vi "runtest format template keys.vi"(0 "Connection Refnum":T11, 1 "POST (empty)":T10, 3 "User Action (Run)":enum16{"Run", "Repeat"}(ring), 5 "Test Sequence ID":string, 9 "Fields / Results":T8, 11 "error in (no error)":errorcluster, 12 "Timer":u32, 13 "User/Station":T1, 14 "Run Permissions":T9) -> (4 "Connection Refnum":T11, 10 "Template Keys":T10, 15 "error out":errorcluster)   [LabVIEW 2011]
uses:
  Addons/internet/utils/keyedarr.llb/Keyed Array.ctl
  SI.LIB/ODBC/SQL Controls/Connection Refnum.ctl
  server/database/Fields/Field Record.ctl
  server/database/Fields/Field DataTypes.ctl
  server/database/Fields/Field NextItem.ctl
  tests/Test Output.ctl
  runtest User - Station.ctl
  server/database/Stations/Instruments/Instrument Record.ctl
  server/database/Stations/Step Associations/Step Association Record.ctl
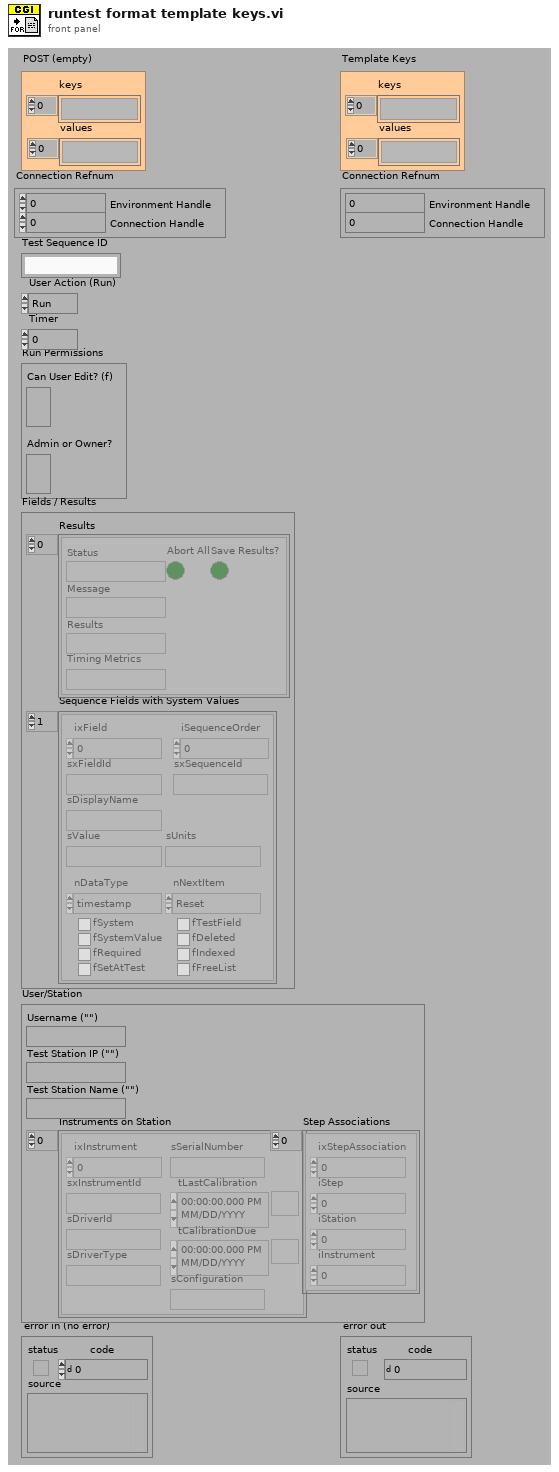
[diagram p1: front panel]
types:
  T1 = typedef "runtest User - Station.ctl" = cluster{"Username (\"\")":string, "Test Station IP (\"\")":string, "Test Station Name (\"\")":string, "Instruments on Station":T2[], "Step Associations":T3[]}
  T2 = typedef "Instrument Record.ctl" = cluster{"ixInstrument":i32, "sxInstrumentId":string, "sDriverId":string, "sDriverType":string, "sSerialNumber":string, "tLastCalibration":timestamp, "tCalibrationDue":timestamp, "sConfiguration":string}
  T3 = typedef "Step Association Record.ctl" = cluster{"ixStepAssociation":i32, "iStep":i32, "iStation":i32, "iInstrument":i32}
  T4 = typedef "Field Record.ctl" = cluster{"ixField":i32, "iSequenceOrder":i32, "sxFieldId":string, "sxSequenceId":string, "sDisplayName":string, "sValue":string, "sUnits":string, "nDataType":T5, "nNextItem":T6, "fSystem":bool, "fSystemValue":bool, "fRequired":bool, "fSetAtTest":bool, "fTestField":bool, "fDeleted":bool, "fIndexed":bool, "fFreeList":bool}
  T5 = typedef "Field DataTypes.ctl" = enum32{"text", "numeric", "list", "timestamp", "boolean"}
  T6 = typedef "Field NextItem.ctl" = enum32{"Reset", "Retain", "Auto-Increment"}
  T7 = typedef "Test Output.ctl" = cluster{"Status":string, "Message":string, "Results":string, "Abort All":bool, "Save Results?":bool, "Timing Metrics":string}
  T8 = cluster{"Sequence Fields with System Values":T4[], "Results":T7[]}
  T9 = cluster{"Can User Edit? (f)":bool, "Admin or Owner?":bool}
  T10 = typedef "Keyed Array.ctl" = cluster{"keys":string[], "values":string[]}
  T11 = typedef "Connection Refnum.ctl" = cluster{"Environment Handle":i32, "Connection Handle":i32}
  T12 = typedef "Sequence Record.ctl" = cluster{"ixSequence":i32, "sxSequenceId":string, "sDescription":string, "sCreator":string, "tCreationDate":timestamp, "sModifier":string, "tModifiedDate":timestamp, "fApproved":bool, "fSpartanSetsSN":bool, "fOverwriteData":bool, "fStopOnFail":bool, "fDisableQuickMode":bool, "fPartialExecution":bool, "fAutoNextItem":bool, "fDoNotPrintOnFail":bool}
  T13 = typedef "Step Record.ctl" = cluster{"ixStep":i32, "sxSequenceId":string, "sxTestId":string, "iIndex":i32, "iRepeat":i32, "iQuickMode":i32, "sTag":string, "sDatasheetsCSV":string, "bConfiguration":string}
  T14 = typedef "Test Record.ctl" = cluster{"ixTest":i32, "sxTestId":string, "sVersion":string, "sDriverTypes":string[], "sDescription":string, "iQuickMode":i32}
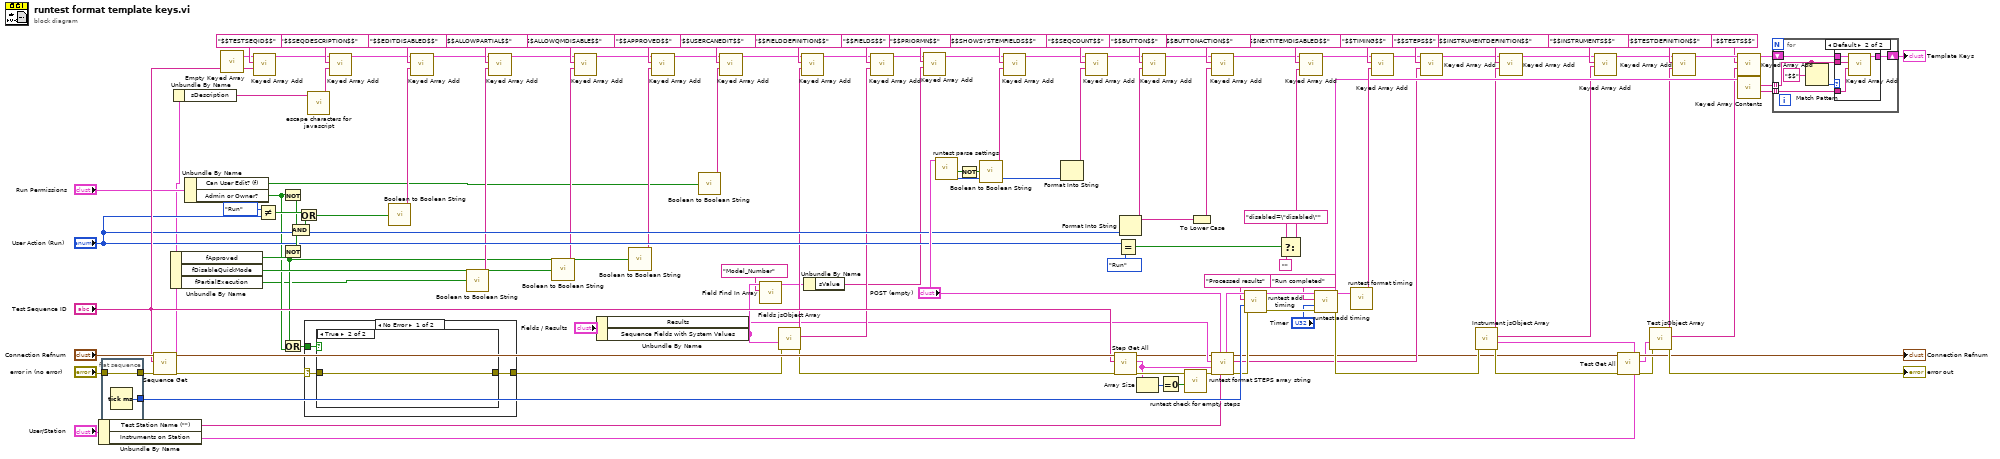
[diagram p0: block diagram]
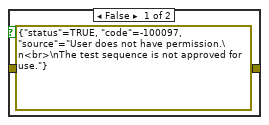
[diagram p2: hidden frame]
diagram:
  n1 = Unbundle By Name("User/Station") -> ("Test Station Name (\"\")"=w2:string, "Instruments on Station"=w26:T2[])
  n2 = flat-sequence {
    tunnel: "error in (no error)" -> [w130]
    tunnel: [w130] -> w79
    tunnel: [w129] -> w78
    frame #0 {
      n3 = Tick Count (ms)() -> (millisecond timer value=w129:u32)
    }
  }
  n4 = call "Sequence Get.vi"("error in (no error)"=w79, "sxSequenceId (\"\")"="Test Sequence ID", "Connection Refnum"="Connection Refnum") -> ("error out"=w45:errorcluster, "Sequence Record"=w31:T12, "Connection Refnum"=w113:T11)  [unwired: 6 out]
  n5 = Unbundle By Name(w31) -> ("fApproved"=w50:bool, "fDisableQuickMode"=w61:bool, "fPartialExecution"=w1:bool)
  n6 = Unbundle By Name(w31) -> ("sDescription"=w30:string)
  n7 = Unbundle By Name("Run Permissions") -> ("Can User Edit? (f)"=w57:bool, "Admin or Owner?"=w49:bool)
  n8 = call "Empty Keyed Array.vi"() -> ("empty keyed array"=w111:T10)  [unwired: 3 out]
  n9 = call "Keyed Array Add.vi"("value"="Test Sequence ID", "key"="$$TESTSEQID$$", "array in"=w111) -> ("array out"=w33:T10)  [unwired: 1 in, 3 out]
  n10 = Not Equal?(x=enum16{"Run", "Repeat"}."Run", y="User Action (Run)") -> (x != y?=w91:bool)
  n11 = Not(x=w49) -> (.not. x?=w88:bool)
  n12 = Not(x=w50) -> (.not. x?=w89:bool)
  n13 = Or(x=w50, y=w49) -> (x .or. y?=w48:bool)
  n14 = And(x=w88, y=w89) -> (x .and. y?=w90:bool)
  n15 = Or(x=w91, y=w90) -> (x .or. y?=w64:bool)
  n16 = case shown="No Error" w45 {
    selector: w45 -> [w131 w136]
    tunnel: w48 -> [w133 _]
    tunnel: [w132 w136] -> w47
    frame No Error {
      n17 = case shown="True" w133 {
        tunnel: [errorcluster {"status"=TRUE, "code"=-100097, "source"="User does not have permission.\n<br>\nThe test sequence is not approved for use."} ("error out") w135] -> w132
        tunnel: w131 -> [_ w135]
        frame False {
        }
        frame True {
        }
      }
    }
    frame Error {
      # "LOGIC at left preempts incoming erro\nsince fApproved will be false"
    }
  }
  n18 = call "escape characters for javascript.vi"("String (\"\")"=w30) -> ("escaped String"=w29:string)  [unwired: 4 in]
  n19 = call "Keyed Array Add.vi"("value"=w29, "key"="$$SEQDESCRIPTION$$", "array in"=w33) -> ("array out"=w32:T10)  [unwired: 1 in, 3 out]
  n20 = call "Boolean to Boolean String.vi"("Boolean"=w64) -> ("Boolean string"=w63:string)  [unwired: 1 in]
  n21 = call "Keyed Array Add.vi"("value"=w63, "key"="$$EDITDISABLED$$", "array in"=w32) -> ("array out"=w46:T10)  [unwired: 1 in, 3 out]
  n22 = call "Boolean to Boolean String.vi"("Boolean"=w1) -> ("Boolean string"=w62:string)  [unwired: 1 in]
  n23 = call "Keyed Array Add.vi"("value"=w62, "key"="$$ALLOWPARTIAL$$", "array in"=w46) -> ("array out"=w106:T10)  [unwired: 1 in, 3 out]
  n24 = call "Boolean to Boolean String.vi"("Boolean"=w61) -> ("Boolean string"=w60:string)  [unwired: 1 in]
  n25 = call "Keyed Array Add.vi"("value"=w60, "key"="$$ALLOWQMDISABLE$$", "array in"=w106) -> ("array out"=w99:T10)  [unwired: 1 in, 3 out]
  n26 = Unbundle By Name("Fields / Results") -> ("Results"=w6:T7[], "Sequence Fields with System Values"=w38:T4[])
  n27 = call "Boolean to Boolean String.vi"("Boolean"=w50) -> ("Boolean string"=w58:string)  [unwired: 1 in]
  n28 = call "Keyed Array Add.vi"("value"=w58, "key"="$$APPROVED$$", "array in"=w99) -> ("array out"=w100:T10)  [unwired: 1 in, 3 out]
  n29 = call "Boolean to Boolean String.vi"("Boolean"=w57) -> ("Boolean string"=w56:string)  [unwired: 1 in]
  n30 = call "Keyed Array Add.vi"("value"=w56, "key"="$$USERCANEDIT$$", "array in"=w100) -> ("array out"=w54:T10)  [unwired: 1 in, 3 out]
  n31 = call "Field Find In Array.vi"("FieldID or Display Name(\"\")"="Model_Number" ("FieldID or Display Name(\"\")"), "Field Array"=w38) -> ("Field"=w36:T4)  [unwired: 1 in, 8 out]
  n32 = call "Fields jsObject Array.vi"("error in (no error)"=w47, "FIELDS (none)"=w38) -> ("error out"=w59:errorcluster, "Fields jsObject Array"=w52:string, "Field jsObject Definition"=w51:string)  [unwired: 2 in, 5 out]
  n33 = call "Keyed Array Add.vi"("value"=w51, "key"="$$FIELDDEFINITION$$", "array in"=w54) -> ("array out"=w53:T10)  [unwired: 1 in, 3 out]
  n34 = Unbundle By Name(w36) -> ("sValue"=w35:string)
  n35 = call "Keyed Array Add.vi"("value"=w52, "key"="$$FIELDS$$", "array in"=w53) -> ("array out"=w40:T10)  [unwired: 1 in, 3 out]
  n36 = call "Keyed Array Add.vi"("value"=w35, "key"="$$PRIORMN$$", "array in"=w40) -> ("array out"=w39:T10)  [unwired: 1 in, 3 out]
  n37 = call "runtest parse settings.vi"("POST (empty)"="POST (empty)") -> ("SeqCount"=w104:i32, "Hide System Fields?"=w44:bool)  [unwired: 9 out]
  n38 = Not(x=w44) -> (.not. x?=w42:bool)
  n39 = call "Boolean to Boolean String.vi"("Boolean"=w42) -> ("Boolean string"=w43:string)  [unwired: 1 in]
  n40 = call "Keyed Array Add.vi"("value"=w43, "key"="$$SHOWSYSTEMFIELDS$$", "array in"=w39) -> ("array out"=w84:T10)  [unwired: 1 in, 3 out]
  n41 = Format Into String(w104) -> (resulting string=w103:string)  [unwired: 3 in, 1 out]
  n42 = call "Keyed Array Add.vi"("value"=w103, "key"="$$SEQCOUNT$$", "array in"=w84) -> ("array out"=w83:T10)  [unwired: 1 in, 3 out]
  n43 = call "Step Get All.vi"("error in (no error)"=w59, "sxSequenceId"="Test Sequence ID", "Connection Refnum"=w113) -> ("error out"=w116:errorcluster, "Sequence Steps"=w7:T13[], "Connection Refnum"=w4:T11)  [unwired: 1 in, 5 out]
  n44 = Equal?(x="User Action (Run)", y=enum16{"Run", "Repeat"}."Run") -> (x = y?=w121:bool)
  n45 = Format Into String("User Action (Run)") -> (resulting string=w95:string)  [unwired: 3 in, 1 out]
  n46 = Array Size(array=w7) -> (size(s)=w108:i32)
  n47 = call "Keyed Array Add.vi"("value"=w95, "key"="$$BUTTON$$", "array in"=w83) -> ("array out"=w97:T10)  [unwired: 1 in, 3 out]
  n48 = Equal To 0?(x=w108) -> (x = 0?=w115:bool)
  n49 = call "runtest check for empty steps.vi"("No Steps? (f)"=w115, "error in (no error)"=w116) -> ("error out"=w86:errorcluster)  [unwired: 9 out]
  n50 = To Lower Case(string=w95) -> (all lower case string=w94:string)
  n51 = call "Keyed Array Add.vi"("value"=w94, "key"="$$BUTTONACTION$$", "array in"=w97) -> ("array out"=w96:T10)  [unwired: 1 in, 3 out]
  n52 = call "runtest format STEPS array string.vi"("sxStationId"=w2, "POST (empty)"="POST (empty)", "error in (no error)"=w86, "Sequence Steps"=w7, "Test Step Outputs"=w6, "Connection Refnum"=w4) -> ("error out"=w77:errorcluster, "STEPS array"=w5:string, "Connection Refnum"=w3:T11, "POST out"=w82:T10)  [unwired: 2 out]
  n53 = call "runtest add timing.vi"("error in (no error)"=w77, "Start Tick, ms (0)"=w78, "Function (\"\")"="Processed results", "POST (empty)"=w82) -> ("error out"=w73:errorcluster, "POST out"=w75:T10)  [unwired: 6 out]
  n54 = Select(t="disabled=\"disabled\"", s=w121, f="") -> (s? t:f=w120:string)
  n55 = call "Keyed Array Add.vi"("value"=w120, "key"="$$NEXTITEMDISABLED$$", "array in"=w96) -> ("array out"=w66:T10)  [unwired: 1 in, 3 out]
  n56 = call "runtest add timing.vi"("error in (no error)"=w73, "Start Tick, ms (0)"="Timer", "Function (\"\")"="Run completed", "POST (empty)"=w75) -> ("error out"=w28:errorcluster, "POST out"=w69:T10)  [unwired: 6 out]
  n57 = call "runtest format timing.vi"("POST (empty)"=w69) -> ("$$TIMING$$"=w76:string)  [unwired: 2 out]
  n58 = call "Keyed Array Add.vi"("value"=w76, "key"="$$TIMING$$", "array in"=w66) -> ("array out"=w87:T10)  [unwired: 1 in, 3 out]
  n59 = call "Keyed Array Add.vi"("value"=w5, "key"="$$STEPS$$", "array in"=w87) -> ("array out"=w22:T10)  [unwired: 1 in, 3 out]
  n60 = call "Instrument jsObject Array.vi"("error in (no error)"=w28, "Instruments (empty)"=w26) -> ("error out"=w11:errorcluster, "Instruments jsObject Array"=w24:string, "Instrument Definition"=w20:string)  [unwired: 2 in, 5 out]
  n61 = call "Keyed Array Add.vi"("value"=w20, "key"="$$INSTRUMENTDEFINITION$$", "array in"=w22) -> ("array out"=w21:T10)  [unwired: 1 in, 3 out]
  n62 = call "Keyed Array Add.vi"("value"=w24, "key"="$$INSTRUMENTS$$", "array in"=w21) -> ("array out"=w15:T10)  [unwired: 1 in, 3 out]
  n63 = call "Test Get All.vi"("error in (no error)"=w11, "Connection Refnum"=w3) -> ("error out"=w9:errorcluster, "Test Records"=w8:T14[], "Connection Refnum"=→"Connection Refnum":T11)  [unwired: 6 in, 1 out]
  n64 = call "Test jsObject Array.vi"("error in (no error)"=w9, "TESTS (none)"=w8) -> ("error out"=→"error out":errorcluster, "Tests jsObject Array"=w13:string, "Test Definition"=w12:string)  [unwired: 7 in]
  n65 = call "Keyed Array Add.vi"("value"=w12, "key"="$$TESTDEFINITION$$", "array in"=w15) -> ("array out"=w19:T10)  [unwired: 1 in, 3 out]
  n66 = call "Keyed Array Add.vi"("value"=w13, "key"="$$TESTS$$", "array in"=w19) -> ("array out"=w16:T10)  [unwired: 1 in, 3 out]
  n67 = call "Keyed Array Contents.vi"("array in"=w69) -> ("values"=w67:string[], "keys"=w68:string[])  [unwired: 5 out]
  n68 = for {
    shift-right: [w141] -> w65
    shift-left: w16 -> [w142]
    tunnel: w68 -> [w140] mode=indexing
    tunnel: w67 -> [w137] mode=indexing
    n69 = Match Pattern(string=w140, regular expression="$$") -> (offset past match=w138:i32)  [unwired: 4 out]
    n70 = case shown="Default" w138 {
      tunnel: w142 -> [w143 w147]
      tunnel: [w143 w146] -> w141
      tunnel: w140 -> [_ w145]
      tunnel: w137 -> [_ w144]
      frame -1 {
      }
      frame Default {
        n71 = call "Keyed Array Add.vi"("value"=w144, "key"=w145, "array in"=w147) -> ("array out"=w146:T10)  [unwired: 1 in, 3 out]
      }
    }
  }
  "Template Keys" <- w65
